vi "Sonar Strafe.vi"(6 "reinitialize? (F)":bool=TRUE, 8 "Sonar Side":string="Sonar Left Side", 9 "Desired Wall Distance":dbl=32.0, 11 "Speed":dbl format="%#_13g") -> (0 "Distance Reached?":bool=TRUE, 1 "Joy Y":dbl, 3 "Joy X":dbl)   [LabVIEW 2014]
uses:
  <vilib>/Rock Robotics/WPI/Ultrasonic/WPI_SonarMB1010AnalogRefNum Registry Get.vi
  <vilib>/Rock Robotics/WPI/Ultrasonic/WPI_SonarMB1010AnalogGetRange.vi
  <vilib>/addons/control/pid/NI_PID_pid.lvlib
  <vilib>/addons/control/pid/pid.llb/PID (DBL).vi
panel:
  in  "Forward Output Range":cluster{"output high":dbl, "output low":dbl}={"output high"=0.75, "output low"=-0.75} {"output low" format="%.2f"; "output high" format="%.2f"}
  in  "Forward PID gains":T1={"proportional gain (Kc)"=0.1, "integral time (Ti, min)"=1.0, "derivative time (Td, min)"=0.0} {"derivative time (Td, min)" format="%.3f"; "integral time (Ti, min)" format="%.3f"; "proportional gain (Kc)" format="%.3f"}
  in  "Forward Range":dbl=0.8
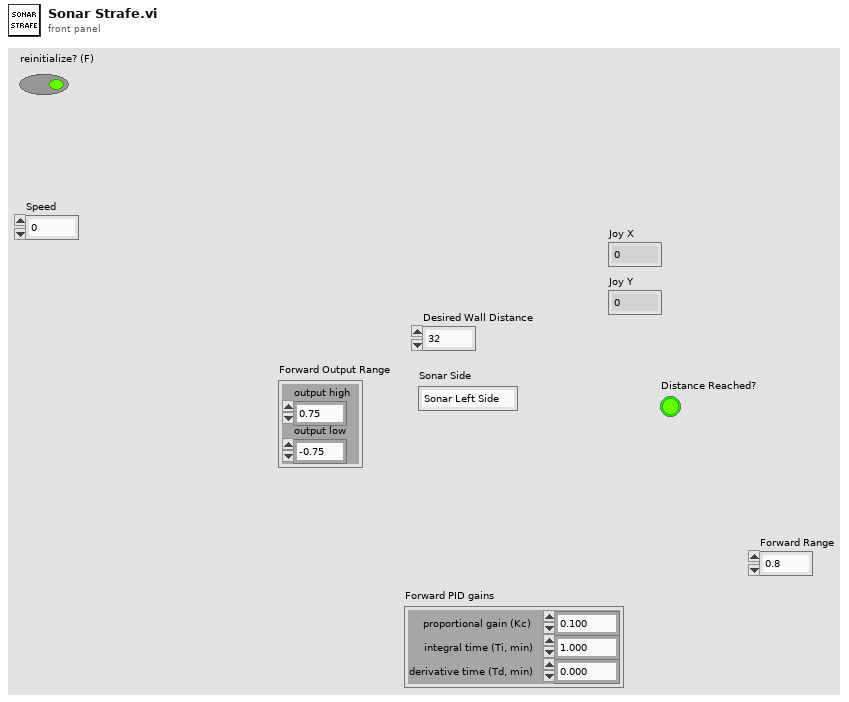
[diagram p1: front panel]
types:
  T1 = cluster{"proportional gain (Kc)":dbl, "integral time (Ti, min)":dbl, "derivative time (Td, min)":dbl}
  T2 = typedef "WPI_SonarMB1010AnalogDeviceRef.ctl" = cluster{"AIDeviceRef":T3, "Scaling factor (V/in)":dbl, "Average Bits":u8}
  T3 = typedef "WPI_AnalogChannelDevRef.ctl" = cluster{"DevStatus":errorcluster, "Controller":T4, "Analog Channel":T5}
  T4 = typedef "FPGA_TypedefAnalogModule.ctl" = enum16{"Controller 1"}
  T5 = typedef "FPGA_AIChannel.ctl" = enum8{"AI 0", "AI 1", "AI 2", "AI 3", "AI MXP 0", "AI MXP 1", "AI MXP 2", "AI MXP 3", "Invalid"}
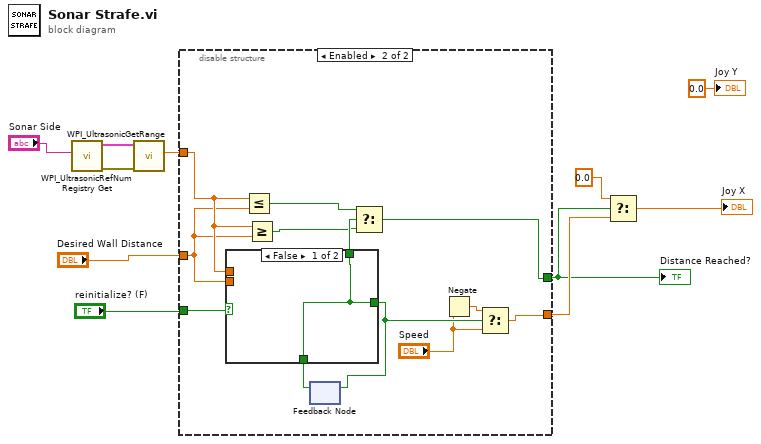
[diagram p0: block diagram]
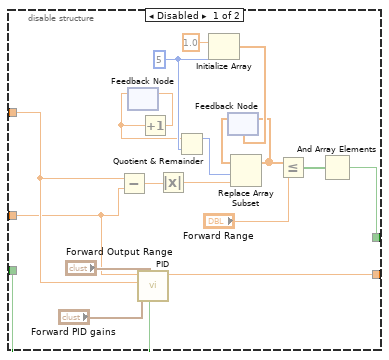
[diagram p2: hidden frame]
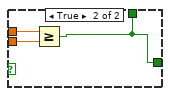
[diagram p3: hidden frame]
diagram:
  n1 = call-poly <vilib>:"WPI_UltrasonicRefNum Registry Get.vi"("refnum name"="Sonar Side") -> ("error out"=w10:errorcluster, "SonarMB1010AnalogDevRef"=w11:T2)  [unwired: 9 in]
  n2 = call-poly <vilib>:"WPI_UltrasonicGetRange.vi"("error in"=w10, "SonarMB1010AnalogDevRef"=w11) -> ("Distance"=w7:dbl)  [unwired: 7 in, 2 out]
  n3 = disable-structure shown="Enabled" {
    disable-tunnel: w7 -> [w26 w39]
    disable-tunnel: "Desired Wall Distance" -> [w25 w38]
    disable-tunnel: [w24 w34] -> w3
    disable-tunnel: [w13 w35] -> w2
    disable-tunnel: "reinitialize? (F)" -> [w12 w41]
    frame Disabled {
      w18 = 5 ("dimension size")
      n4 = Subtract(x=w26, y=w25) -> (x-y=w30:dbl)
      n5 = feedback #1() -> (w16:dbl)  [unwired: 1 in]
      n6 = call-poly <vilib>:"PID.vi"("reinitialize? (F)"=w12, "output range"="Forward Output Range", "PID gains"="Forward PID gains", "process variable"=w26, "setpoint"=w25) -> ("output"=w24:dbl)  [unwired: 5 in, 1 out]
      n7 = Increment(x=w16) -> (x+1=w19:dbl)
      n8 = feedback-in #1(w19) -> ()
      n9 = Absolute Value(x=w30) -> (abs(x)=w20:dbl)
      n10 = Quotient & Remainder(x=w16, y=w18) -> (x-y*floor(x/y)=w17:i32)  [unwired: 1 out]
      n11 = Initialize Array(1.0 ("element"), w18) -> (w22:dbl[])
      n12 = feedback #2(w22) -> (w21:dbl[])
      n13 = Replace Array Subset(array=w21, new element=w20, index=w17) -> (w15:dbl[])
      n14 = feedback-in #2(w15) -> ()
      n15 = Less Or Equal?(x=w15, y="Forward Range") -> (x <= y?=w14:bool[])
      n16 = And Array Elements(Boolean array=w14) -> (logical AND=w13:bool)
    }
    frame Enabled {
      n17 = Less Or Equal?(x=w39, y=w38) -> (x <= y?=w42:bool)
      n18 = Greater Or Equal?(x=w39, y=w38) -> (x >= y?=w37:bool)
      n19 = feedback #3() -> (w36:bool)  [unwired: 1 in]
      n20 = case shown="False" w41 {
        tunnel: w39 -> [_ w46]
        tunnel: w38 -> [_ w45]
        tunnel: [w43 w44] -> w40
        tunnel: [w43 w44] -> w33
        tunnel: w36 -> [w43 _]
        frame False {
        }
        frame True {
          n21 = Greater Or Equal?(x=w46, y=w45) -> (x >= y?=w44:bool)
        }
      }
      n22 = feedback-in #3(w33) -> ()
      n23 = Select(t=w42, s=w40, f=w37) -> (s? t:f=w35:bool)
      n24 = Negate(x="Speed") -> (-x=w32:dbl)
      n25 = Select(t=w32, s=w33, f="Speed") -> (s? t:f=w34:dbl)
    }
  }
  "Distance Reached?" <- w2
  n26 = Select(t=0.0, s=w2, f=w3) -> (s? t:f=→"Joy X":dbl)
  "Joy Y" <- 0.0 ("Joy Y")
